vi "TickCount.vi"() -> ()   [LabVIEW 2019]
panel:
  out "x-y":u32
  in  "stop":bool
  in  "OK Button":bool
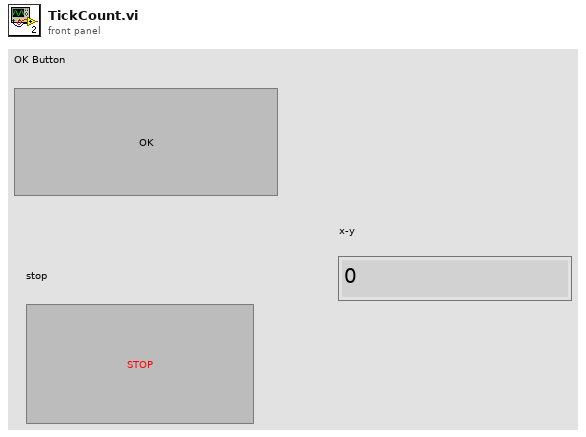
[diagram p1: front panel]
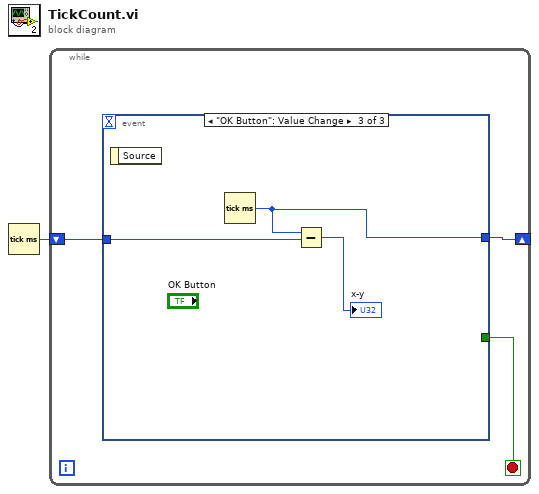
[diagram p0: block diagram]
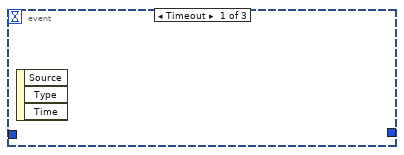
[diagram p2: hidden frame]
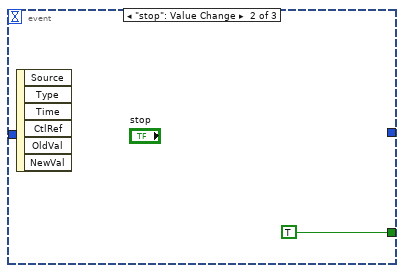
[diagram p3: hidden frame]
diagram:
  n1 = Tick Count (ms)() -> (millisecond timer value=w1:u32)
  n2 = while {
    shift-right: [w3] -> _
    shift-left: w1 -> [w2]
    stop <- w4 stop-if-true
    n3 = event shown="[2] \"OK Button\": Value Change" {
      selector: _ -> [_ _ _]
      dyn-events: _ -> [_ _ _]
      timeout: _ -> [_ _ _]
      tunnel: [_ TRUE _] -> w4
      tunnel: [_ _ w7] -> w3
      tunnel: w2 -> [_ _ w8]
      event Timeout {
        n4 = event-data() -> ()  [unwired: 1 in, 3 out]
      }
      event "stop": Value Change {
        n5 = event-data() -> ()  [unwired: 1 in, 6 out]
      }
      event "OK Button": Value Change {
        n6 = event-data() -> ()  [unwired: 1 in, 1 out]
        n7 = Tick Count (ms)() -> (millisecond timer value=w7:u32)
        n8 = Subtract(x=w7, y=w8) -> (x-y=→"x-y":u32)
      }
    }
  }
